vi "Tree_ArrayHierarchicalPath_Tests.vi"(11 "error in":errorcluster) -> (15 "error out":errorcluster)   [LabVIEW 2016, in "DronaTest.lvlib"]
uses:
  DronaTest.lvlib
  APIs/Stimulus/ControlValue/SetValueAuto.vi
  APIs/Stimulus/ControlValue/Controls/Tree/SetValueByHierarchicalPathArray.vi
  APIs/Assert/AssertControlValue/Equal.vi
  <vilib>/addons/_JKI Toolkits/Caraya/classes/Test/Test.lvclass
  Drona.lvlib
  <vilib>/SLL Toolkit/SLL Debug/SLL Debug.lvlib
  APIs/Assert/AssertControlValue/AssertControlValue.lvlib
  APIs/Stimulus/ControlValue/ControlValue.lvlib
  <vilib>/addons/_JKI Toolkits/Caraya/classes/Assert/Assert.lvclass
  APIs/Stimulus/ControlValue/Controls/Tree/StimulusTree.lvlib
  APIs/Get/GetControlRef/GetControlRef.lvlib
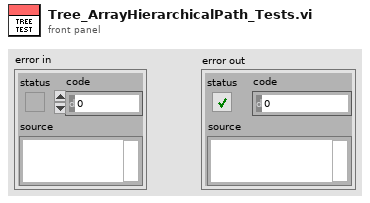
[diagram p1: front panel]
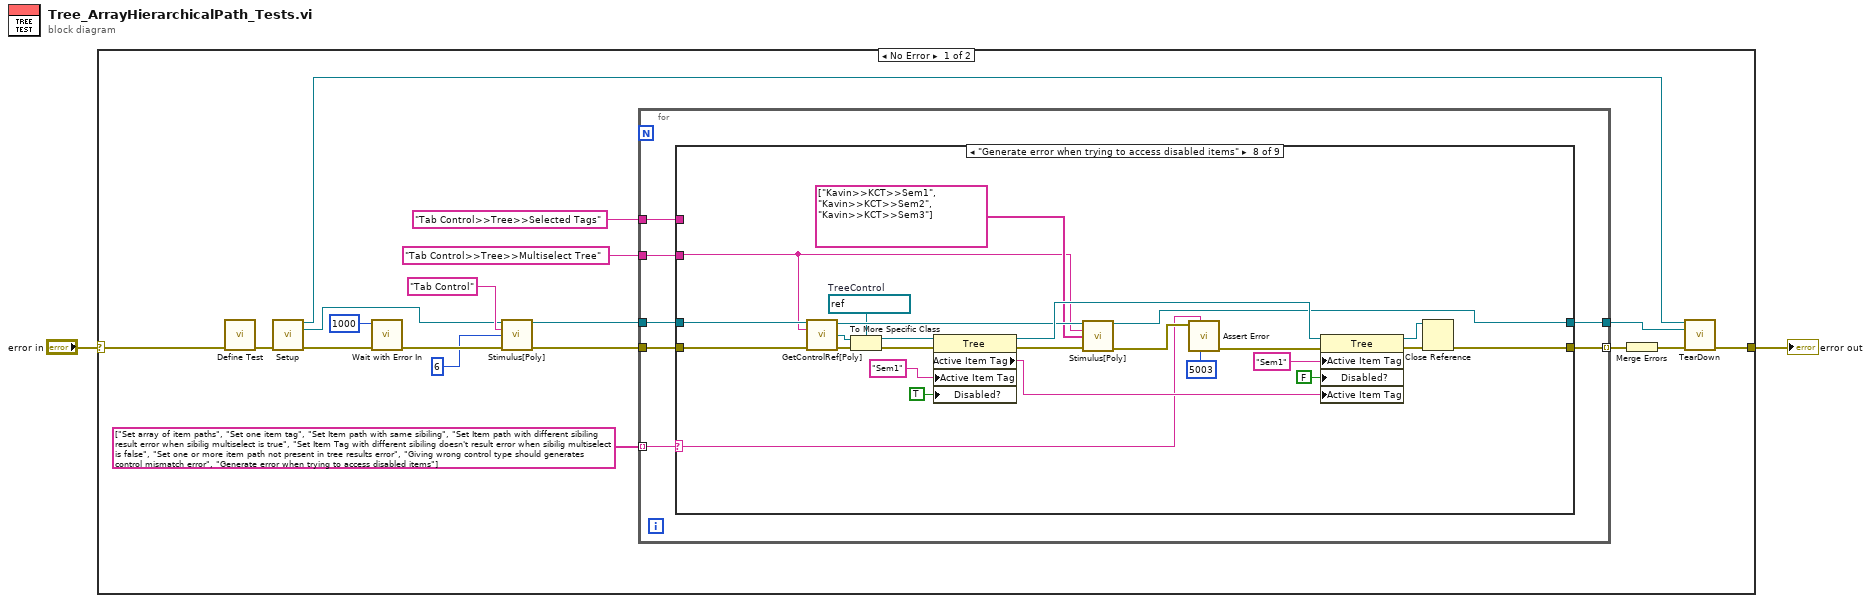
[diagram p0: block diagram]
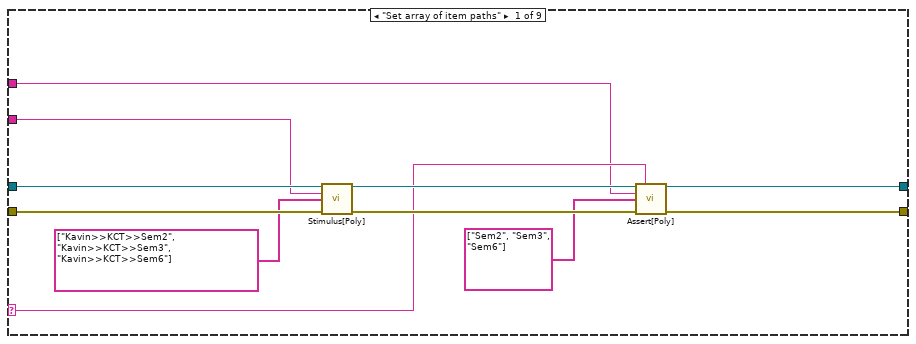
[diagram p2: hidden frame]
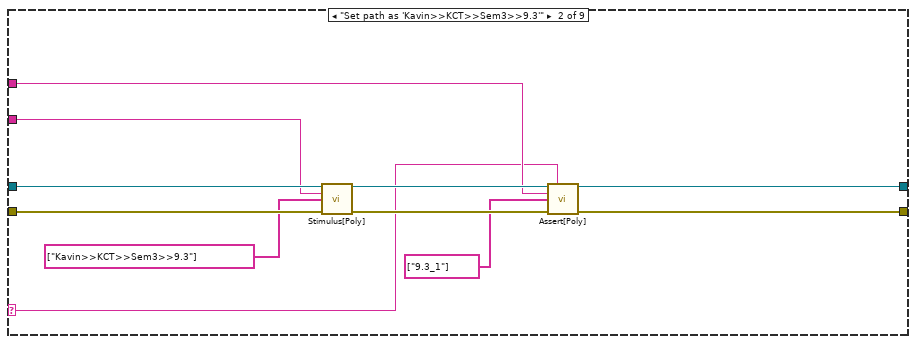
[diagram p3: hidden frame]
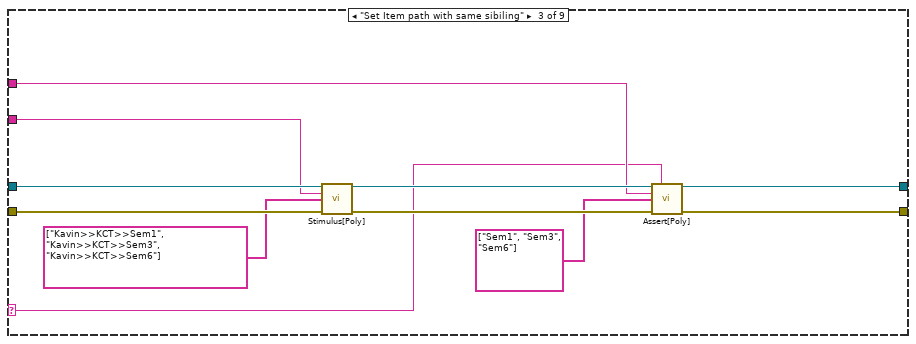
[diagram p4: hidden frame]
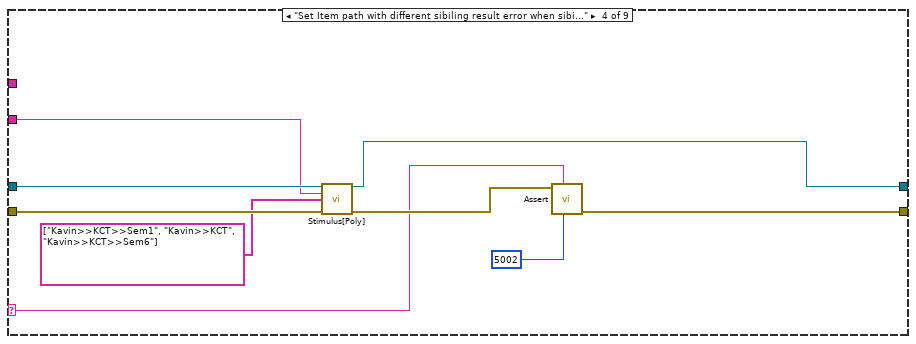
[diagram p5: hidden frame]
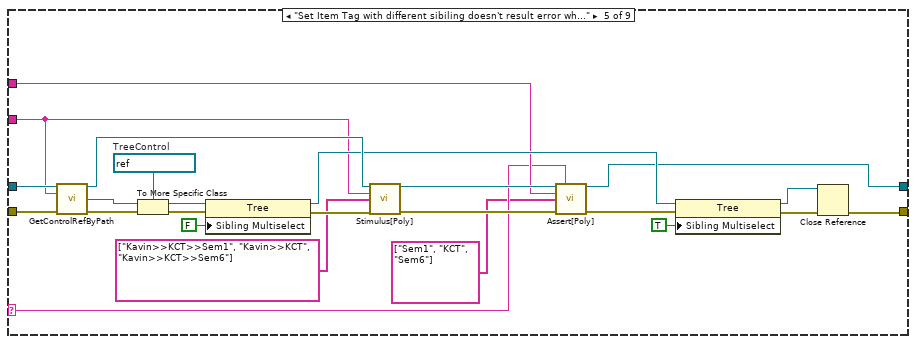
[diagram p6: hidden frame]
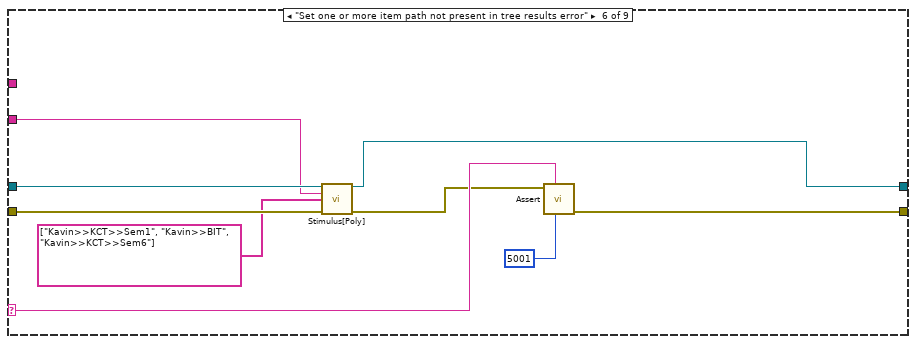
[diagram p7: hidden frame]
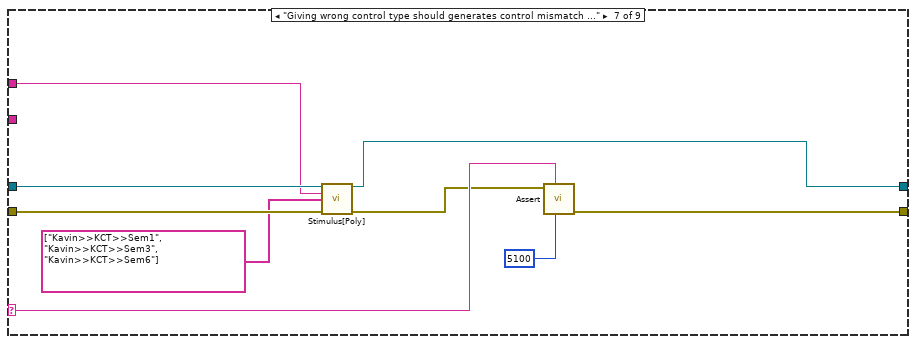
[diagram p8: hidden frame]
diagram:
  n1 = case shown="No Error" "error in" {
    selector: "error in" -> [w20 w139]
    tunnel: [w3 w139] -> w1
    frame No Error {
      n2 = call <vilib>:"Define Test.vi"("error in (no error)"=w20) -> ("error out"=w9:errorcluster)  [unwired: 9 in, 1 out]
      n3 = call "Setup.vi"("error in"=w9) -> ("Application Ref"=w4:refnum<vi>, "VI out"=w8:refnum<vi>, "error out"=w7:errorcluster)  [unwired: 12 in]
      n4 = call <vilib>:"Wait with Error In.vi"("error in (no error)"=w7, "milliseconds to wait"=u32 1000) -> ("error out"=w18:errorcluster)  [unwired: 9 in]
      n5 = call-poly "Stimulus[Poly].vi"("VI Reference In"=w8, "Control Path"="Tab Control", "Value (Signaling)"=6, "error in"=w18) -> ("VI Reference Out"=w14:refnum<vi>, "error out"=w17:errorcluster)  [unwired: 10 in]
      n6 = for {
        tunnel: w14 -> [w26]
        tunnel: "Tab Control>>Tree>>Multiselect Tree" ("Control Path") -> [w25]
        tunnel: "Tab Control>>Tree>>Selected Tags" ("Control Path") -> [w24]
        tunnel: string[] ["Set array of item paths", "Set one item tag", "Set Item path with same sibiling", "Set Item path with different sibiling result error when sibilig multiselect is true", "Set Item Tag with different sibiling doesn't result error when sibilig multiselect is false", "Set one or more item path not present in tree results error", "Giving wrong control type should generates control mismatch error", "Generate error when trying to access disabled items"] -> [w22] mode=indexing
        tunnel: [w21] -> w5
        tunnel: w17 -> [w27]
        tunnel: [w23] -> w10 mode=indexing
        n7 = case shown="\"Generate error when trying to access disabled items\"" w22 {
          selector: w22 -> [w32 w41 w52 w63 w75 w99 w108 w113 _]
          tunnel: w27 -> [w38 w49 w60 w69 w78 w102 w111 w117 w138]
          tunnel: w26 -> [w37 w48 w59 w68 w77 w101 w110 w116 w137]
          tunnel: w25 -> [w30 w45 w56 w67 w70 w94 _ w112 _]
          tunnel: w24 -> [w31 w44 w55 _ w76 _ w104 _ _]
          tunnel: [w34 w43 w54 w66 w73 w100 w109 w115 w138] -> w23
          tunnel: [w33 w42 w53 w65 w74 w98 w107 w114 w137] -> w21
          frame "Set array of item paths" {
            n8 = call-poly "Stimulus[Poly].vi"("VI Reference In"=w37, "Control Path"=w30, "Hierarchical Path Array"=string[] ["Kavin>>KCT>>Sem2", "Kavin>>KCT>>Sem3", "Kavin>>KCT>>Sem6"], "Error In"=w38) -> ("VI Reference Out"=w35:refnum<vi>, "Error Out"=w36:errorcluster)  [unwired: 10 in]
            n9 = call-poly "Assert[Poly].vi"("VI Reference In"=w35, "Test Label"=w32, "Control Path"=w31, "Control Value"=string[] ["Sem2", "Sem3", "Sem6"], "Error In"=w36) -> ("VI Reference Out"=w33:refnum<vi>, "Error Out"=w34:errorcluster)  [unwired: 8 in, 1 out]
          }
          frame "Set path as 'Kavin>>KCT>>Sem3>>9.3'" {
            n10 = call-poly "Stimulus[Poly].vi"("VI Reference In"=w48, "Control Path"=w45, "Hierarchical Path Array"=string[] ["Kavin>>KCT>>Sem3>>9.3"] ("Item Name"), "Error In"=w49) -> ("VI Reference Out"=w46:refnum<vi>, "Error Out"=w47:errorcluster)  [unwired: 10 in]
            n11 = call-poly "Assert[Poly].vi"("VI Reference In"=w46, "Test Label"=w41, "Control Path"=w44, "Control Value"=string[] ["9.3_1"], "Error In"=w47) -> ("VI Reference Out"=w42:refnum<vi>, "Error Out"=w43:errorcluster)  [unwired: 8 in, 1 out]
          }
          frame "Set Item path with same sibiling" {
            n12 = call-poly "Stimulus[Poly].vi"("VI Reference In"=w59, "Control Path"=w56, "Hierarchical Path Array"=string[] ["Kavin>>KCT>>Sem1", "Kavin>>KCT>>Sem3", "Kavin>>KCT>>Sem6"], "Error In"=w60) -> ("VI Reference Out"=w57:refnum<vi>, "Error Out"=w58:errorcluster)  [unwired: 10 in]
            n13 = call-poly "Assert[Poly].vi"("VI Reference In"=w57, "Test Label"=w52, "Control Path"=w55, "Control Value"=string[] ["Sem1", "Sem3", "Sem6"], "Error In"=w58) -> ("VI Reference Out"=w53:refnum<vi>, "Error Out"=w54:errorcluster)  [unwired: 8 in, 1 out]
          }
          frame "Set Item path with different sibiling result error when sibilig multiselect is true" {
            n14 = call-poly "Stimulus[Poly].vi"("VI Reference In"=w68, "Control Path"=w67, "Hierarchical Path Array"=string[] ["Kavin>>KCT>>Sem1", "Kavin>>KCT", "Kavin>>KCT>>Sem6"], "Error In"=w69) -> ("VI Reference Out"=w65:refnum<vi>, "Error Out"=w64:errorcluster)  [unwired: 10 in]
            n15 = call-poly <vilib>:"Assert.vi"("error code (1)"=5002, "Label"=w63, "Error?"=w64) -> ("error out"=w66:errorcluster)  [unwired: 7 in, 1 out]
          }
          frame "Set Item Tag with different sibiling doesn't result error when sibilig multiselect is false" {
            w88 = refnum<vi> refnum  # TreeControl
            n16 = call "GetControlRefByPath.vi"("VI Reference In"=w77, "Control Path"=w70, "error In"=w78) -> ("VI Reference Out"=w91:refnum<vi>, "Ctl Refnum"=w90:refnum<vi>, "error out"=w89:errorcluster)  [unwired: 10 in]
            n17 = To More Specific Class(target class=w88, reference=w90, error in=w89) -> (specific class reference=w87:refnum<vi>, error out=w86:errorcluster)
            n18 = property class="Tree"(reference=w87, error in=w86, "Sibling Multiselect"=FALSE) -> (reference out=w80:refnum<vi>, error out=w84:errorcluster)
            n19 = call-poly "Stimulus[Poly].vi"("VI Reference In"=w91, "Control Path"=w70, "Hierarchical Path Array"=string[] ["Kavin>>KCT>>Sem1", "Kavin>>KCT", "Kavin>>KCT>>Sem6"], "Error In"=w84) -> ("VI Reference Out"=w92:refnum<vi>, "Error Out"=w93:errorcluster)  [unwired: 10 in]
            n20 = call-poly "Assert[Poly].vi"("VI Reference In"=w92, "Test Label"=w75, "Control Path"=w76, "Control Value"=string[] ["Sem1", "KCT", "Sem6"], "Error In"=w93) -> ("VI Reference Out"=w74:refnum<vi>, "Error Out"=w82:errorcluster)  [unwired: 8 in, 1 out]
            n21 = property class="Tree"(reference=w80, error in=w82, "Sibling Multiselect"=TRUE) -> (reference out=w79:refnum<vi>, error out=w81:errorcluster)
            n22 = Close Reference(reference=w79, error in (no error)=w81) -> (error out=w73:errorcluster)
          }
          frame "Set one or more item path not present in tree results error" {
            n23 = call-poly "Stimulus[Poly].vi"("VI Reference In"=w101, "Control Path"=w94, "Hierarchical Path Array"=string[] ["Kavin>>KCT>>Sem1", "Kavin>>BIT", "Kavin>>KCT>>Sem6"], "Error In"=w102) -> ("VI Reference Out"=w98:refnum<vi>, "Error Out"=w97:errorcluster)  [unwired: 10 in]
            n24 = call-poly <vilib>:"Assert.vi"("error code (1)"=5001, "Label"=w99, "Error?"=w97) -> ("error out"=w100:errorcluster)  [unwired: 7 in, 1 out]
          }
          frame "Giving wrong control type should generates control mismatch error" {
            n25 = call-poly "Stimulus[Poly].vi"("VI Reference In"=w110, "Control Path"=w104, "Hierarchical Path Array"=string[] ["Kavin>>KCT>>Sem1", "Kavin>>KCT>>Sem3", "Kavin>>KCT>>Sem6"], "Error In"=w111) -> ("VI Reference Out"=w107:refnum<vi>, "Error Out"=w106:errorcluster)  [unwired: 10 in]
            n26 = call-poly <vilib>:"Assert.vi"("error code (1)"=5100, "Label"=w108, "Error?"=w106) -> ("error out"=w109:errorcluster)  [unwired: 7 in, 1 out]
          }
          frame "Generate error when trying to access disabled items" {
            w122 = refnum<vi> refnum  # TreeControl
            n27 = call-poly "GetControlRef[Poly].vi"("VI Reference In"=w116, "Control Path"=w112, "error In"=w117) -> ("VI Reference Out"=w129:refnum<vi>, "Ctl Refnum"=w121:refnum<vi>, "error out"=w119:errorcluster)  [unwired: 10 in]
            n28 = To More Specific Class(target class=w122, reference=w121, error in=w119) -> (specific class reference=w123:refnum<vi>, error out=w120:errorcluster)
            n29 = property class="Tree"(reference=w123, error in=w120, "Active Item Tag"="Sem1" ("Active Item:Tag"), "Disabled?"=TRUE ("Active Item:Disabled?")) -> (reference out=w133:refnum<vi>, error out=w128:errorcluster, "Active Item Tag"=w134:string)
            n30 = call-poly "Stimulus[Poly].vi"("VI Reference In"=w129, "Control Path"=w112, "Hierarchical Path Array"=string[] ["Kavin>>KCT>>Sem1", "Kavin>>KCT>>Sem2", "Kavin>>KCT>>Sem3"] ("Item Tags Array"), "Error In"=w128) -> ("VI Reference Out"=w114:refnum<vi>, "Error Out"=w130:errorcluster)  [unwired: 10 in]
            n31 = call <vilib>:"Assert Error.vi"("error code (1)"=5003, "Label"=w113, "Error?"=w130) -> ("error out"=w131:errorcluster)  [unwired: 7 in, 1 out]
            n32 = property class="Tree"(reference=w133, error in=w131, "Active Item Tag"="Sem1" ("Active Item:Tag"), "Disabled?"=FALSE ("Active Item:Disabled?"), "Active Item Tag"=w134) -> (reference out=w127:refnum<vi>, error out=w126:errorcluster)
            n33 = Close Reference(reference=w127, error in (no error)=w126) -> (error out=w115:errorcluster)
          }
          frame Default {
          }
        }
      }
      n34 = Merge Errors(w10) -> (w6:errorcluster)
      n35 = call "TearDown.vi"("Application Ref"=w4, "VI in"=w5, "error in (no error)"=w6) -> ("error out"=w3:errorcluster)  [unwired: 12 in]
    }
    frame Error {
    }
  }
  "error out" <- w1
